vi "get used disk space.vi"(8 "error in (no error)":errorcluster, 10 "image path":path, 11 "Simulated Camera in":refnum<class "Simulated Camera.lvclass">) -> (0 "error out":errorcluster, 3 "Simulated Camera out":refnum<class "Simulated Camera.lvclass">)   [LabVIEW 2018, in "Simulated Camera.lvclass"]
uses:
  Simulated Camera.lvclass
  Simulated Camera.lvclass/Simulated Camera.ctl
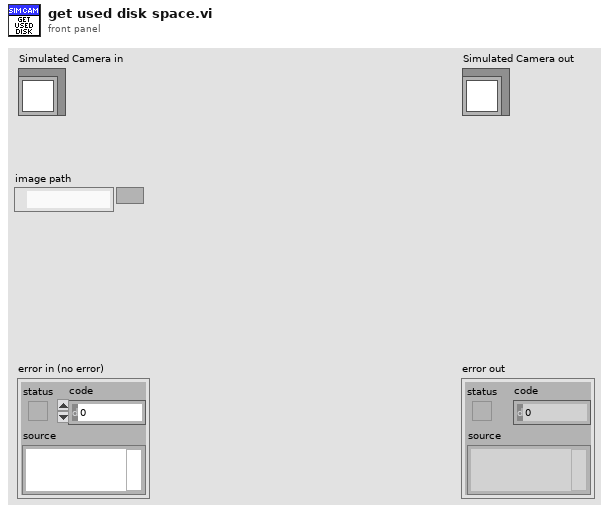
[diagram p1: front panel]
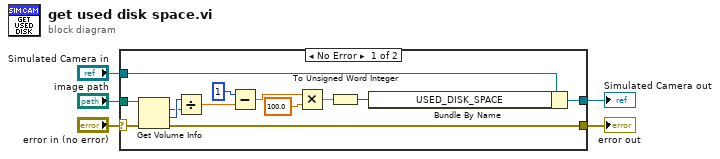
[diagram p0: block diagram]
diagram:
  n1 = case shown="No Error" "error in (no error)" {
    selector: "error in (no error)" -> [w17 w20]
    tunnel: [w16 w20] -> w4
    tunnel: [w18 w19] -> w2
    tunnel: "Simulated Camera in" -> [w7 w19]
    tunnel: "image path" -> [w6 _]
    frame No Error {
      n2 = Get Volume Info(8:w17, 11:w6) -> (0:w16:errorcluster, 1:w15:i64, 2:w14:i64)  [unwired: 3 out]
      n3 = Divide(x=w15, y=w14) -> (x/y=w13:dbl)
      n4 = Subtract(x=1, y=w13) -> (x-y=w11:dbl)
      n5 = Multiply(x=w11, y=100.0) -> (x*y=w9:dbl)
      n6 = To Unsigned Word Integer(number=w9) -> (unsigned 16bit integer=w8:u16)
      n7 = Bundle By Name(cluster=w7, "USED_DISK_SPACE"=w8) -> (w18:refnum<class "Simulated Camera.lvclass">)
    }
    frame Error {
    }
  }
  "error out" <- w4
  "Simulated Camera out" <- w2
